vi "util.time.calc.vi"(11 "Begin Time":T1 caption="Open" format="ON:    %<%H:%M>T") -> (3 "daily seconds counter":i32)   [LabVIEW 2024]
uses:
  controls/UiScheduleTimestamp.ctl
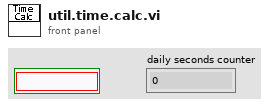
[diagram p1: front panel]
types:
  T1 = typedef "UiScheduleTimestamp.ctl" = timestamp
  T2 = typedef "LVDateTimeRec.ctl" = cluster{"fractional second":dbl, "second":i32, "minute":i32, "hour":i32, "day of month":i32, "month":i32, "year":i32, "day of week":i32, "day of year":i32, "DST":i32}
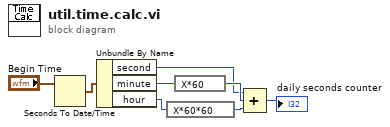
[diagram p0: block diagram]
diagram:
  n1 = Seconds To Date/Time(time stamp (now)="Begin Time") -> (date time rec=w7:T2)  [unwired: 1 in]
  n2 = Unbundle By Name(w7) -> ("second"=w1:i32, "minute"=w5:i32, "hour"=w6:i32)
  n3 = expression code="X*60*60"(w6) -> (w4:i32)
  n4 = expression code="X*60"(w5) -> (w2:i32)
  n5 = Compound Arithmetic op=ADD(w1, w2, w4) -> (→"daily seconds counter":i32)
